vi "PromptUserForAttributeValues.vi"(11 "Name of Command":string) -> (3 "Attributes":string[][](array[string]))   [LabVIEW 2017]
panel:
  out "Array 2":u32[](array[numeric])
  out "Control Value:Get All":cluster{"Name":string, "Variant Data":variant}[](array[cluster])
  in  "vi path":path=path "C:/Users/Bendethic/Desktop/AutoRoutineCreator/TestCommands/DriveForDistance.vi"
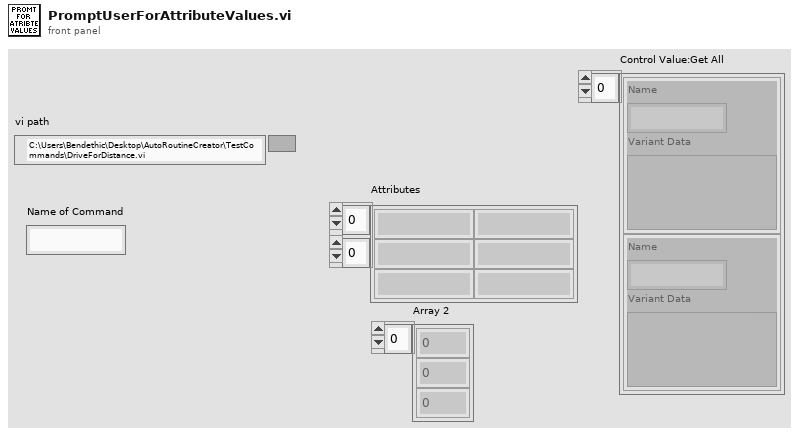
[diagram p1: front panel]
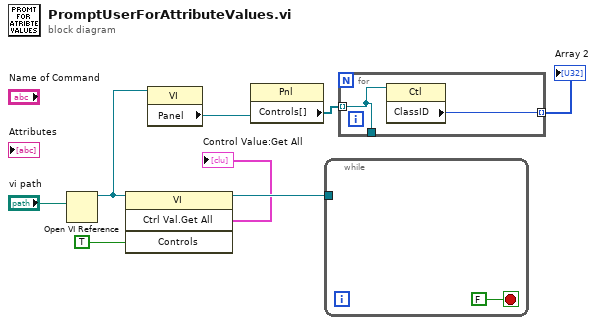
[diagram p0: block diagram]
diagram:
  n1 = Open VI Reference(vi path="vi path") -> (vi reference=w4:refnum<vi>)  [unwired: 5 in, 1 out]
  n2 = invoke class="VI" method="Ctrl Val.Get All"(reference=w4, "Controls"=TRUE) -> (reference out=w7:refnum<vi>, "Get All Control Values Variant"=→"Control Value:Get All":cluster{"Name":string, "Variant Data":variant}[])  [unwired: 2 in, 2 out]
  n3 = property class="VI"(reference=w4) -> ("Panel"=w1:refnum<vi>)  [unwired: 1 in, 2 out]
  n4 = property class="Pnl"(reference=w1) -> ("Controls[]"=w3:refnum<vi>[])  [unwired: 1 in, 2 out]
  n5 = while {
    tunnel: w7 -> [_]
    stop <- FALSE stop-if-true
  }
  n6 = for {
    tunnel: w3 -> [w10] mode=indexing
    tunnel: [w11] -> w2 mode=indexing
    tunnel: [w10] -> _
    n7 = property class="Ctl"(reference=w10) -> ("ClassID"=w11:u32)  [unwired: 1 in, 2 out]
  }
  "Array 2" <- w2
